vi "Initialize.vi"(8 "error in":errorcluster, 11 "Plugin_Driver in":refnum<class "Plugin_Driver.lvclass">) -> (0 "error out":errorcluster, 3 "Plugin_Driver out":refnum<class "Plugin_Driver.lvclass">)   [LabVIEW 2020, in "Plugin.lvlib" / "Plugin_Driver.lvclass"]
doc: "This VI is a wrapper API for Instrumnet Driver's Initialize API."
uses:
  Plugin_Driver.lvclass
  Drivers/Instrument Driver/Instrument Driver.lvclass
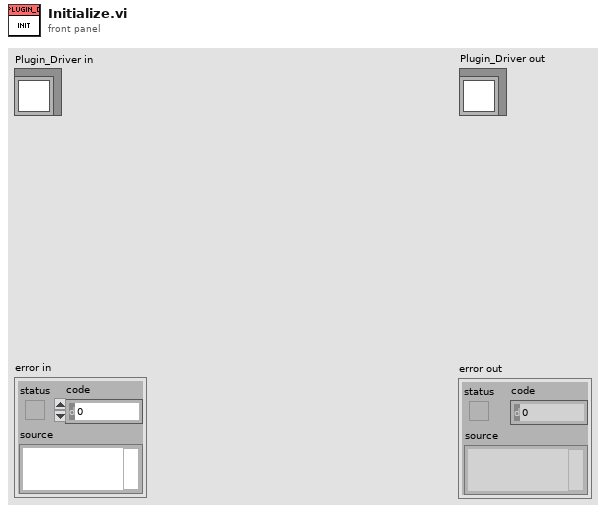
[diagram p1: front panel]
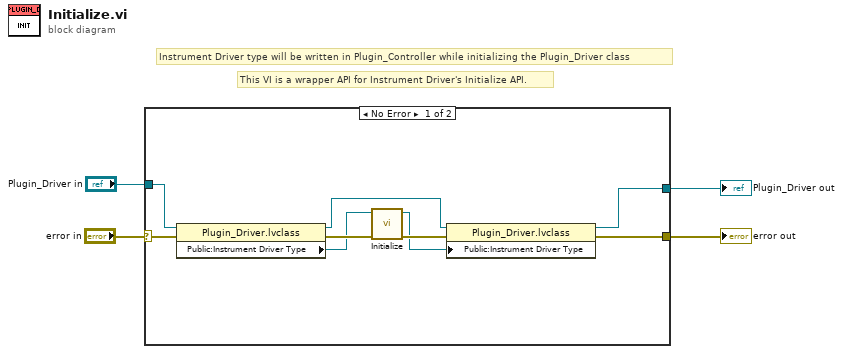
[diagram p0: block diagram]
diagram:
  # "This VI is a wrapper API for Instrument Driver's Initialize API."
  # "Instrument Driver type will be written in Plugin_Controller while initializing the Plugin_Driver class"
  n1 = case shown="No Error" "error in" {
    selector: "error in" -> [w9 w15]
    tunnel: [w12 w15] -> w3
    tunnel: [w11 w14] -> w2
    tunnel: "Plugin_Driver in" -> [w10 w14]
    frame No Error {
      n2 = property class="Plugin_Driver.lvclass"(reference=w10, error in=w9) -> (reference out=w6:refnum<class "Plugin_Driver.lvclass">, error out=w8:errorcluster, "Public:Instrument Driver Type"=w7:refnum<class "Instrument Driver.lvclass">)
      n3 = call-dynamic "Initialize.vi"("error in"=w8, "Instrument Driver in"=w7) -> ("error out"=w13:errorcluster, "Instrument Driver out"=w5:refnum<class "Instrument Driver.lvclass">)  [unwired: 8 in]
      n4 = property class="Plugin_Driver.lvclass"(reference=w6, error in=w13, "Public:Instrument Driver Type"=w5) -> (reference out=w11:refnum<class "Plugin_Driver.lvclass">, error out=w12:errorcluster)
    }
    frame Error {
    }
  }
  "error out" <- w3
  "Plugin_Driver out" <- w2
